vi "parse.list.vi"(9 "div end":string, 10 "div start":string, 11 "body":string) -> (3 "list array":string[](array[string]))   [LabVIEW 2024, in "comic_class.lvclass"]
uses:
  comic_class.lvclass
  comic_class.lvclass/comic_class.ctl
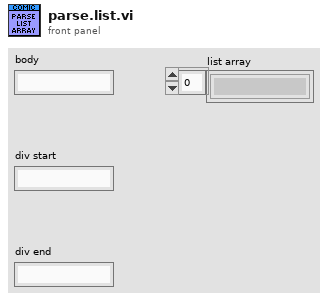
[diagram p1: front panel]
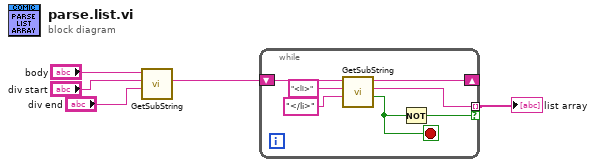
[diagram p0: block diagram]
diagram:
  n1 = call "GetSubString.vi"("End Search"="div end", "Start Search"="div start", "String In"="body") -> ("Match"=w2:string)  [unwired: 6 in, 2 out]
  n2 = while {
    shift-right: [w9] -> _
    shift-left: w2 -> [w12]
    tunnel: [w8] -> w1 mode=indexing if=w6
    stop <- w7 stop-if-true
    n3 = call "GetSubString.vi"("End Search"="</li>", "Start Search"="<li>", "String In"=w12) -> ("Not Found?"=w7:bool, "Match"=w8:string, "Following String Out"=w9:string)  [unwired: 6 in]
    n4 = Not(x=w7) -> (.not. x?=w6:bool)
  }
  "list array" <- w1
